vi "GOOPUtil_GenericCreate.vi"(0 "GOOP Class Path":path, 1 "Control Names":string[](array[string]), 2 "Control Values":variant[](array[variant]), 5 "error in (no error)":errorcluster) -> (12 "GOOP constructor VI ref":refnum<vi>, 14 "GOOP Object":refnum<class>, 19 "error out":errorcluster)   [LabVIEW 2016, in "GOOPUtility.lvlib"]
doc: "Creates an instance of the GOOP class specified by the path. The path could either be directly to the constructor method, the .lvclass file or to the class folder. It is also possible to set the constructor input parameters by the \"Control Names\" and \"Control Values\" inputs.\n\nThe output \"GOOP constructor VI ref\" is a reference to the constructor VI, don't close this reference until the object is destroyed. It will prevent the LabVIEW garbage collector to unload the constructor from memory.\n\nSometimes it is also necessary to set the constructor as \"reentrant execution - share clones between instances\", else the VI might not be able to run using VI server.\n\nThis is a collection of generic GOOP utility VIs. Please notice that it is important that the frontpanel of the Create, Destroy and GetObjectStatus is not removed when building an application."
uses:
  <vilib>/addons/GOOPUtility/GOOPUtility.lvlib
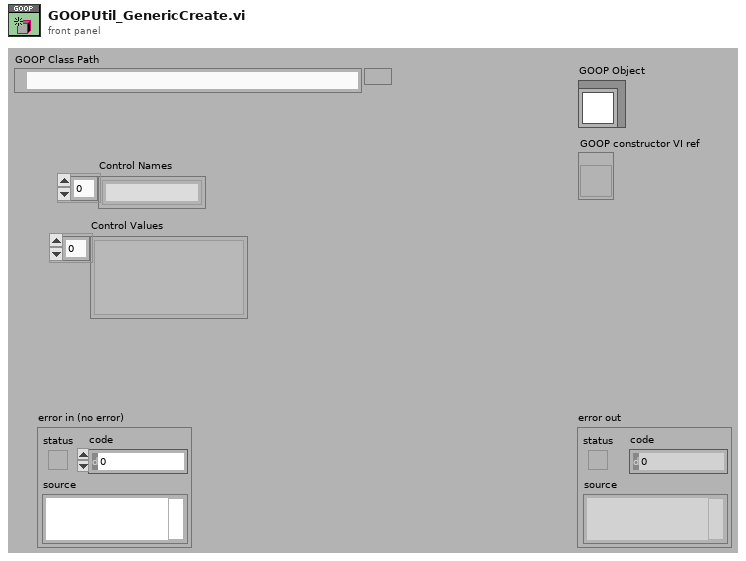
[diagram p1: front panel]
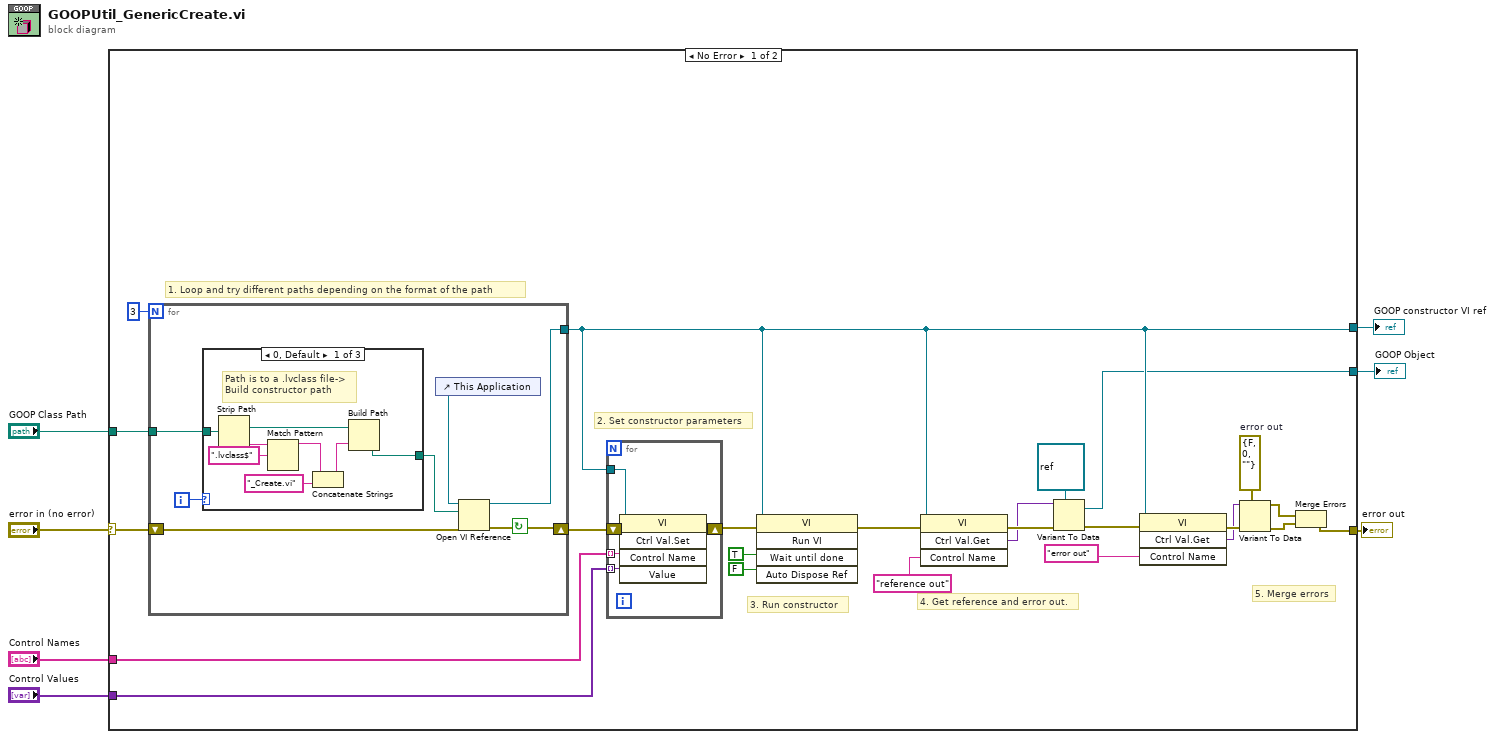
[diagram p0: block diagram]
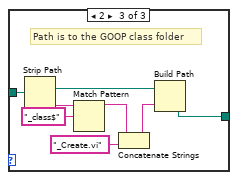
[diagram p3: hidden frame]
diagram:
  n1 = case shown="No Error" "error in (no error)" {
    selector: "error in (no error)" -> [w31 w60]
    tunnel: [w10 w60] -> w6
    tunnel: "GOOP Class Path" -> [w29 _]
    tunnel: [w16 _] -> w4
    tunnel: "Control Names" -> [w27 _]
    tunnel: "Control Values" -> [w26 _]
    tunnel: [w15 _] -> w1
    frame No Error {
      w11 = errorcluster {"status"=FALSE, "code"=0, "source"=""}  # error out
      # "5. Merge errors"
      # "4. Get reference and error out."
      # "3. Run constructor"
      # "2. Set constructor parameters"
      # "1. Loop and try different paths depending on the format of the path"
      n2 = for {
        N: 3 -> [_]
        shift-right: [w37] -> w28
        shift-left: w31 -> [w41]
        tunnel: w29 -> [w42]
        tunnel: [w40] -> w16
        i -> [w43]
        stop <- w37 continue-if-true
        n3 = case shown="0, Default" w43 {
          tunnel: w42 -> [w51 w52 w53]
          tunnel: [w44 w52 w54] -> w38
          frame 0, Default {
            # "Path is to a .lvclass file->\nBuild constructor path"
            n4 = Strip Path(path=w51) -> (stripped path=w45:path, name=w50:string)
            n5 = Match Pattern(string=w50, regular expression=".lvclass$") -> (before substring=w48:string)  [unwired: 1 in, 3 out]
            n6 = Concatenate Strings(w48, "_Create.vi" ("string")) -> (w46:string)
            n7 = Build Path(base path=w45, name or relative path=w46) -> (appended path=w44:path)
          }
          frame 1 {
            # "Path is directly to constructor."
          }
          frame 2 {
            # "Path is to the GOOP class folder"
            n8 = Strip Path(path=w53) -> (name=w59:string)  [unwired: 1 out]
            n9 = Match Pattern(string=w59, regular expression="_class$") -> (before substring=w57:string)  [unwired: 1 in, 3 out]
            n10 = Concatenate Strings(w57, "_Create.vi" ("string")) -> (w55:string)
            n11 = Build Path(base path=w53, name or relative path=w55) -> (appended path=w54:path)
          }
        }
        n12 = control-ref of="This Application"() -> (w39:refnum<vi>)
        n13 = Open VI Reference(application reference (local)=w39, vi path=w38, error in (no error)=w41) -> (vi reference=w40:refnum<vi>, error out=w37:errorcluster)  [unwired: 3 in]
      }
      n14 = for {
        shift-right: [w32] -> w25
        shift-left: w28 -> [w36]
        tunnel: w16 -> [w35]
        tunnel: w27 -> [w34] mode=indexing
        tunnel: w26 -> [w33] mode=indexing
        n15 = invoke class="VI" method="Ctrl Val.Set"(reference=w35, error in=w36, "Control Name"=w34, "Value"=w33) -> (error out=w32:errorcluster)  [unwired: 1 in, 4 out]
      }
      n16 = invoke class="VI" method="Run VI"(reference=w16, error in=w25, "Wait until done"=TRUE ("Wait Until Done"), "Auto Dispose Ref"=FALSE ("Auto Dispose Reference")) -> (error out=w22:errorcluster)  [unwired: 1 in, 4 out]
      n17 = invoke class="VI" method="Ctrl Val.Get"(reference=w16, error in=w22, "Control Name"="reference out") -> (error out=w20:errorcluster, "Get Control Value Variant"=w19:variant)  [unwired: 1 in, 2 out]
      n18 = Variant To Data(error in=w20, type=refnum<class> refnum ("LabVIEW Object"), Variant=w19) -> (data=w15:refnum<class>, error out=w18:errorcluster)
      n19 = invoke class="VI" method="Ctrl Val.Get"(reference=w16, error in=w18, "Control Name"="error out") -> (error out=w13:errorcluster, "Get Control Value Variant"=w12:variant)  [unwired: 1 in, 2 out]
      n20 = Variant To Data(error in=w13, type=w11, Variant=w12) -> (data=w8:errorcluster, error out=w9:errorcluster)
      n21 = Merge Errors(w8, w9) -> (w10:errorcluster)
    }
    frame Error {
    }
  }
  "error out" <- w6
  "GOOP Object" <- w1
  "GOOP constructor VI ref" <- w4
